vi "GetHeader.vi"(8 "error in (no error)":errorcluster caption="에러 입력(에러 없음)", 11 "ABFFIO 입력":refnum<class "ABFFIO.lvclass">) -> (0 "error out":errorcluster caption="에러 출력", 3 "ABFFIO 출력":refnum<class "ABFFIO.lvclass">)   [LabVIEW 2017, in "ABFFIO.lvclass"]
uses:
  ABFFIO.lvclass
  ABFFIO.lvclass/ABFFIO.ctl
panel:
  out "Header":T1
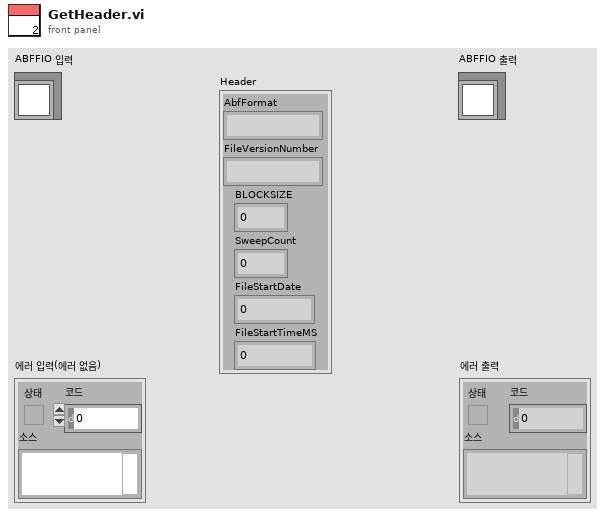
[diagram p1: front panel]
types:
  T1 = cluster{"AbfFormat":string, "FileVersionNumber":string, "BLOCKSIZE":u32, "SweepCount":u32, "FileStartDate":u32, "FileStartTimeMS":u32}
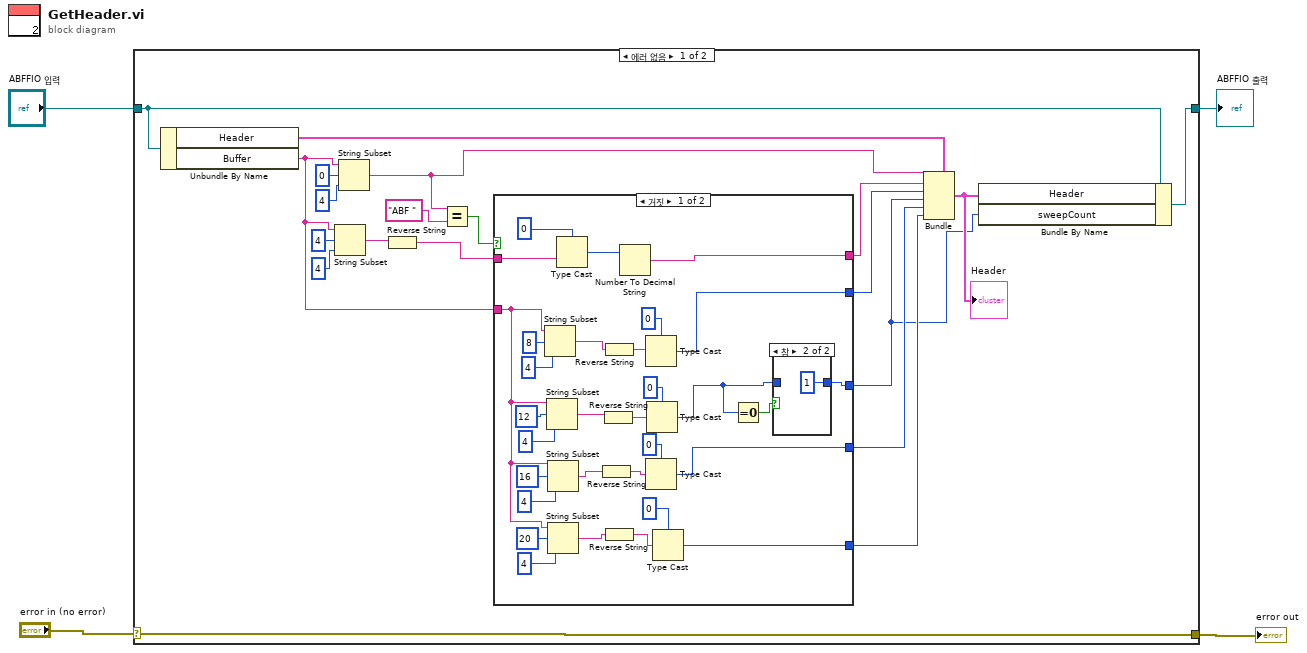
[diagram p0: block diagram]
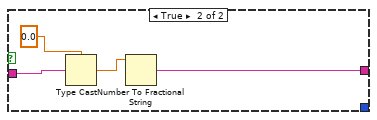
[diagram p3: hidden frame]
diagram:
  n1 = case shown="에러 없음" "error in (no error)" {
    selector: "error in (no error)" -> [w24 w63]
    tunnel: [w24 w63] -> w3
    tunnel: [w20 w62] -> w1
    tunnel: "ABFFIO 입력" -> [w21 w62]
    frame No Error {
      n2 = Unbundle By Name(w21) -> ("Header"=w12:T1, "Buffer"=w13:string)
      n3 = String Subset(string=w13, offset (0)=4 ("오프셋(0)"), length (rest)=4 ("오프셋(0)")) -> (substring=w17:string)
      n4 = String Subset(string=w13, offset (0)=0 ("오프셋(0)"), length (rest)=4 ("오프셋(0)")) -> (substring=w11:string)
      n5 = Reverse String(1:w17) -> (0:w6:string)
      n6 = Equal?(x=w11, y="ABF ") -> (x = y?=w16:bool)
      n7 = case shown="거짓" w16 {
        tunnel: w6 -> [w55 w60]
        tunnel: [w52 w58] -> w10
        tunnel: w13 -> [w32 _]
        tunnel: [w36 _] -> w9
        tunnel: [w25 _] -> w5
        tunnel: [w35 _] -> w8
        tunnel: [w28 _] -> w7
        frame False {
          n8 = String Subset(string=w32, offset (0)=8 ("오프셋(0)"), length (rest)=4 ("길이(나머지)")) -> (substring=w37:string)
          n9 = String Subset(string=w32, offset (0)=12 ("오프셋(0)"), length (rest)=4 ("길이(나머지)")) -> (substring=w48:string)
          n10 = String Subset(string=w32, offset (0)=16 ("오프셋(0)"), length (rest)=4 ("길이(나머지)")) -> (substring=w50:string)
          n11 = String Subset(string=w32, offset (0)=20 ("오프셋(0)"), length (rest)=4 ("길이(나머지)")) -> (substring=w31:string)
          n12 = Type Cast(type=i8 0 ("오프셋(0)"), x=w55) -> (*(type *) &x=w53:i8)
          n13 = Reverse String(1:w50) -> (0:w51:string)
          n14 = Reverse String(1:w48) -> (0:w49:string)
          n15 = Reverse String(1:w37) -> (0:w47:string)
          n16 = Reverse String(1:w31) -> (0:w29:string)
          n17 = Number To Decimal String(number=w53) -> (decimal integer string=w52:string)  [unwired: 1 in]
          n18 = Type Cast(type=u32 0 ("오프셋(0)"), x=w47) -> (*(type *) &x=w36:u32)
          n19 = Type Cast(type=u32 0 ("오프셋(0)"), x=w51) -> (*(type *) &x=w35:u32)
          n20 = Type Cast(type=u32 0 ("오프셋(0)"), x=w49) -> (*(type *) &x=w26:u32)
          n21 = Type Cast(type=u32 0 ("오프셋(0)"), x=w29) -> (*(type *) &x=w28:u32)
          n22 = Equal To 0?(x=w26) -> (x = 0?=w27:bool)
          n23 = case shown="참" w27 {
            tunnel: w26 -> [w56 _]
            tunnel: [w56 u32 1 ("오프셋(0)")] -> w25
            frame False {
            }
            frame True {
            }
          }
        }
        frame True {
          n24 = Type Cast(type=sgl 0.0 ("오프셋(0)"), x=w60) -> (*(type *) &x=w59:sgl)
          n25 = Number To Fractional String(number=w59) -> (F-format string=w58:string)  [unwired: 3 in]
        }
      }
      n26 = Bundle(cluster=w12, "AbfFormat"=w11, "FileVersionNumber"=w10, "BLOCKSIZE"=w9, "SweepCount"=w5, "FileStartDate"=w8, "FileStartTimeMS"=w7) -> (w14:T1)
      "Header" <- w14
      n27 = Bundle By Name(cluster=w21, "Header"=w14, "sweepCount"=w5) -> (w20:refnum<class "ABFFIO.lvclass">)
    }
    frame Error {
    }
  }
  "error out" <- w3
  "ABFFIO 출력" <- w1
